vi "PMBus Get Alert.vi"(9 "PMBusIndex":i32, 10 "DevIndex":i32, 11 "DevType":i32) -> (2 "function return":i32, 3 "pAlertFlag":u8)   [LabVIEW 2010, in "ControlPMBus.lvlib"]
doc: "int WINAPI PMBus_GetAlert(int DevType,int DevIndex,int PMBusIndex,unsigned char *pAlertFlag);"
uses:
  ControlPMBus.lvlib
  ControlPMBus/Ginkgo_Driver.dll
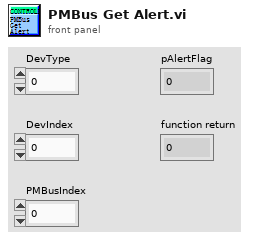
[diagram p1: front panel]
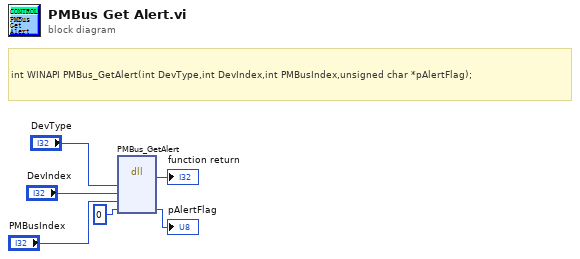
[diagram p0: block diagram]
diagram:
  # "int WINAPI PMBus_GetAlert(int DevType,int DevIndex,int PMBusIndex,unsigned char *pAlertFlag);"
  n1 = dll-call lib="E:/Project/vt_ginkgo/truck/Ginkgo Driver/vs2010/Ginkgo_USB-I2C&SPI&CAN_API_v2.0.3.3/lib/labview_32bit/ControlPMBus/Ginkgo_Driver.*" fn="PMBus_GetAlert"("DevType"="DevType", "DevIndex"="DevIndex", "PMBusIndex"="PMBusIndex", "pAlertFlag"=u8 0) -> (→"function return":i32, "pAlertFlag"=→"pAlertFlag":u8)  [unwired: 6 in, 2 out]
